vi "PID Online (Relay Feedback).vi"(8 "Period":dbl format="%.2f", 9 "Noise level (e)":dbl, 10 "Output amplitude (a)":dbl format="%.2f", 11 "Relay Input amplitude (d)":dbl) -> (1 "Ultimate Frequency (Wo)":dbl, 2 "Ultimate Period (Tu)":dbl, 3 "Ultimate Gain (Ku)":dbl)   [LabVIEW 2017]
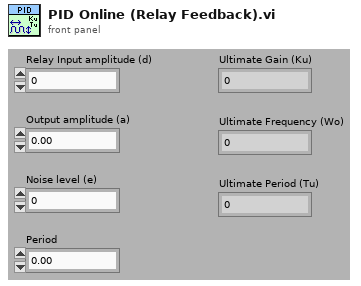
[diagram p1: front panel]
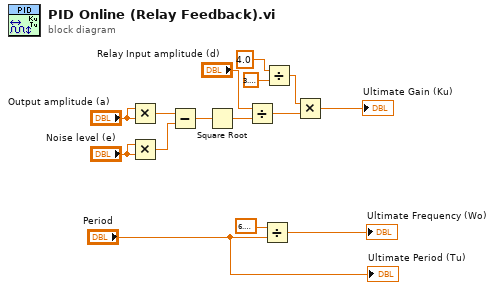
[diagram p0: block diagram]
diagram:
  n1 = Multiply(x="Output amplitude (a)", y="Output amplitude (a)") -> (x*y=w4:dbl)
  n2 = Multiply(x="Noise level (e)", y="Noise level (e)") -> (x*y=w7:dbl)
  n3 = Subtract(x=w4, y=w7) -> (x-y=w6:dbl)
  n4 = Square Root(x=w6) -> (sqrt(x)=w5:dbl)
  n5 = Divide(x="Relay Input amplitude (d)", y=w5) -> (x/y=w3:dbl)
  n6 = Divide(x=6.283185307179586, y="Period") -> (x/y=→"Ultimate Frequency (Wo)":dbl)
  n7 = Divide(x=4.0, y=3.141592653589793) -> (x/y=w11:dbl)
  n8 = Multiply(x=w11, y=w3) -> (x*y=→"Ultimate Gain (Ku)":dbl)
  "Ultimate Period (Tu)" <- "Period"
